vi "StartAcquisitionWithEvent_DEPRECATED.vi"(8 "error in (no error)":errorcluster, 11 "reference in":refnum<class "Camera_IMAQdx.lvclass">) -> (0 "error out":errorcluster, 2 "Frame Complete Event":refnum<event-registration>, 3 "reference out":refnum<class "Camera_IMAQdx.lvclass">)   [LabVIEW 2017, in "Camera_IMAQdx.lvclass"]
doc: "Starts IMAQdx Acquisition and returns the event reference for the Frame Complete Event. Use this with GetCompletedFrame when the Frame Complete Event is fired."
uses:
  Camera_IMAQdx.lvclass
  <vilib>/vision/driver/NI_Vision_Acquisition_Software.lvlib
  <vilib>/vision/driver/IMAQdx.llb/IMAQdx Acquisition Mode.ctl
  <vilib>/userdefined/High Color/IMAQdx.ctl
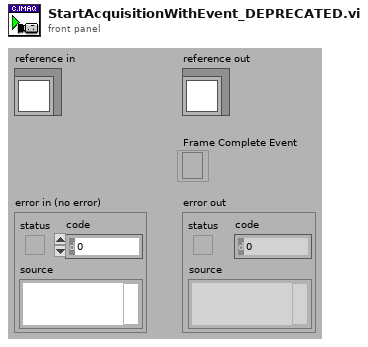
[diagram p1: front panel]
types:
  T1 = typedef "NI_Vision_Acquisition_Software.lvlib/IMAQdx Acquisition Mode.ctl" = enum32{"One Shot", "Continuous"}
  T2 = typedef "Camera_IMAQdx.lvclass/Configuration--Cluster.ctl" = cluster{"Camera Interface Name":string, "Number of Buffers":u32, "Image Name":string, "Image Type":T3}
  T3 = typedef "Image Type" = u32
  T4 = typedef "IMAQdx.ctl" = refnum<k21>
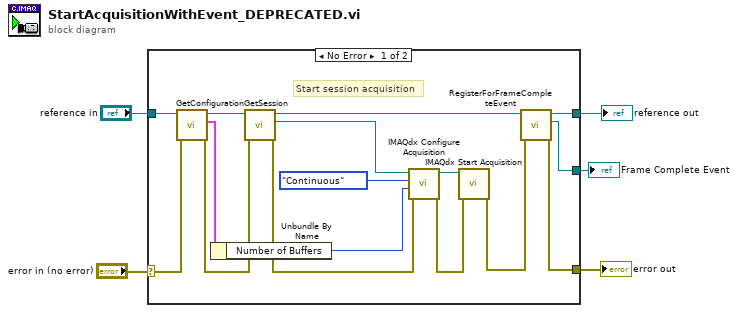
[diagram p0: block diagram]
diagram:
  n1 = case shown="No Error" "error in (no error)" {
    selector: "error in (no error)" -> [w15 w23]
    tunnel: [w7 w23] -> w4
    tunnel: [w9 w22] -> w2
    tunnel: "reference in" -> [w21 w22]
    tunnel: [w6 _] -> w1
    frame No Error {
      # "Start session acquisition"
      n2 = call-dynamic "GetConfiguration.vi"("error in (no error)"=w15, "reference in"=w21) -> ("error out"=w14:errorcluster, "Configuration"=w13:T2, "reference out"=w16:refnum<class "Camera_IMAQdx.lvclass">)  [unwired: 7 in]
      n3 = Unbundle By Name(w13) -> ("Number of Buffers"=w12:u32)
      n4 = call "GetSession.vi"("error in (no error)"=w14, "reference in"=w16) -> ("error out"=w11:errorcluster, "Session"=w19:T4, "reference out"=w20:refnum<class "Camera_IMAQdx.lvclass">)  [unwired: 7 in]
      n5 = call <vilib>:"IMAQdx Configure Acquisition.vi"("error in"=w11, "Number of Buffers"=w12, "Continuous?"=IMAQdx_Acquisition_Mode."Continuous", "Session In"=w19) -> ("error out"=w10:errorcluster, "Session Out"=w18:T4)  [unwired: 6 in]
      n6 = call <vilib>:"IMAQdx Start Acquisition.vi"("error in"=w10, "Session In"=w18) -> ("error out"=w8:errorcluster)  [unwired: 8 in, 1 out]
      n7 = call "RegisterForFrameCompleteEvent.vi"("error in (no error)"=w8, "reference in"=w20) -> ("error out"=w7:errorcluster, "Frame Complete Event"=w6:refnum<event-registration>, "reference in"=w9:refnum<class "Camera_IMAQdx.lvclass">)  [unwired: 7 in]
    }
    frame Error {
    }
  }
  "error out" <- w4
  "reference out" <- w2
  "Frame Complete Event" <- w1
